vi "UI.vi"   [LabVIEW 2018]
uses:
  User Interface/UI.lvclass
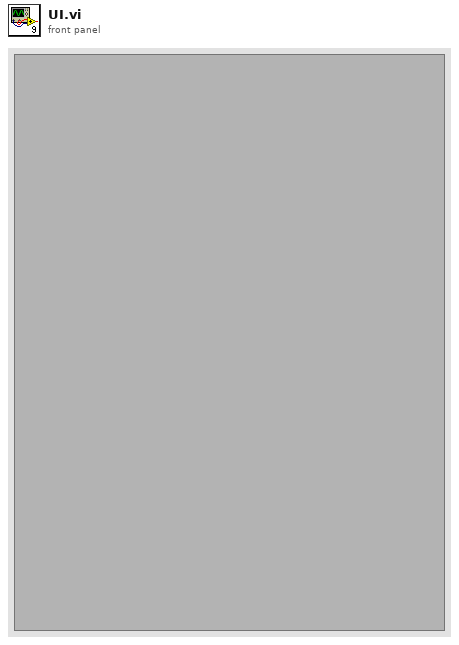
[diagram p1: front panel]
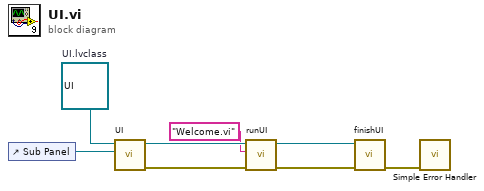
[diagram p0: block diagram]
diagram:
  w8 = refnum<class "UI.lvclass"> refnum  # UI.lvclass
  n1 = control-ref of="Sub Panel"() -> (w7:refnum<vi>)
  n2 = call "UI.vi"("subPanel"=w7, "UI in"=w8) -> ("error out"=w1:errorcluster, "UI out"=w4:refnum<class "UI.lvclass">)  [unwired: 8 in]
  n3 = call "runUI.vi"("error in (no error)"=w1, "Embedded VI"="Welcome.vi" ("First Embedded VI"), "UI in"=w4) -> ("error out"=w5:errorcluster, "UI out"=w3:refnum<class "UI.lvclass">)  [unwired: 7 in]
  n4 = call "finishUI.vi"("error in (no error)"=w5, "UI in"=w3) -> ("error out"=w6:errorcluster)  [unwired: 9 in]
  n5 = call <vilib>:"Simple Error Handler.vi"("error in (no error)"=w6) -> ()  [unwired: 4 in, 5 out]
